vi "libCreate C Array.vi"() -> ()   [LabVIEW 2011]
panel:
  out "concatenated string":string
  in  "String":string
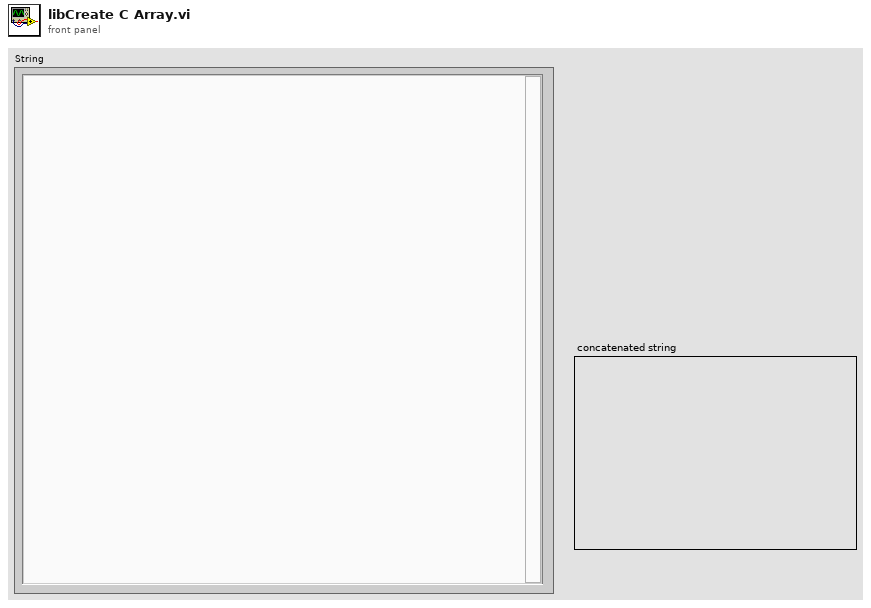
[diagram p1: front panel]
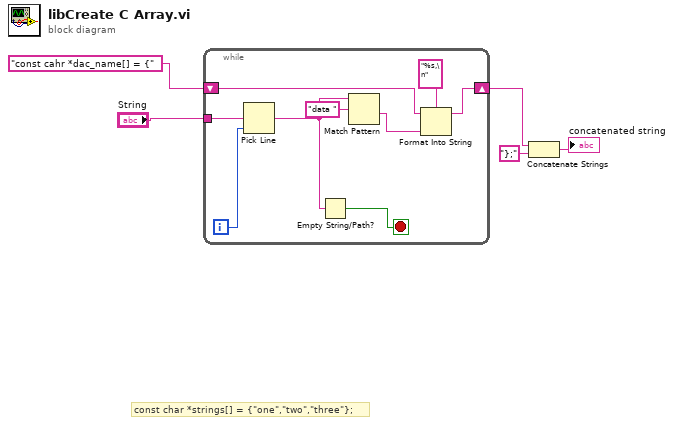
[diagram p0: block diagram]
diagram:
  # "const char *strings[] = {\"one\",\"two\",\"three\"};"
  n1 = while {
    tunnel: "String" -> [w14]
    shift-right: [w10] -> w2
    shift-left: "const cahr *dac_name[] = {" -> [w6]
    i -> [w8]
    stop <- w13 stop-if-true
    n2 = Pick Line(multi-line string=w14, line index=w8) -> (output string=w12:string)  [unwired: 1 in]
    n3 = Empty String/Path?(string/path=w12) -> (empty?=w13:bool)
    n4 = Match Pattern(string=w12, regular expression="data ") -> (after substring=w7:string)  [unwired: 1 in, 3 out]
    n5 = Format Into String(format string="%s,\n", initial string=w6, w7) -> (resulting string=w10:string)  [unwired: 1 in, 1 out]
  }
  n6 = Concatenate Strings(w2, "};" ("string")) -> (→"concatenated string":string)
